vi "Reg Ref.vi"(7 "Tag":T1, 8 "error in (no error)":errorcluster caption="错误输入（无错误）", 11 "User Event Collection 输入":refnum<class "User Event Collection.lvclass"> caption="DNL_LabVIEW Object in") -> (0 "error out":errorcluster caption="错误输出", 2 "Event Registration Refnum":T2, 3 "User Event Collection 输出":refnum<class "User Event Collection.lvclass"> caption="DNL_LabVIEW Object out")   [LabVIEW 2013, in "User Event Collection.lvclass"]
uses:
  User Event Collection.lvclass
  <resource>/importtools/Common/Event/Data Type/Event Registeration Refnum.ctl
  Tag.ctl
  User Event Collection.lvclass/User Event Collection.ctl
  <resource>/importtools/Common/Event/NISAST Event.lvclass
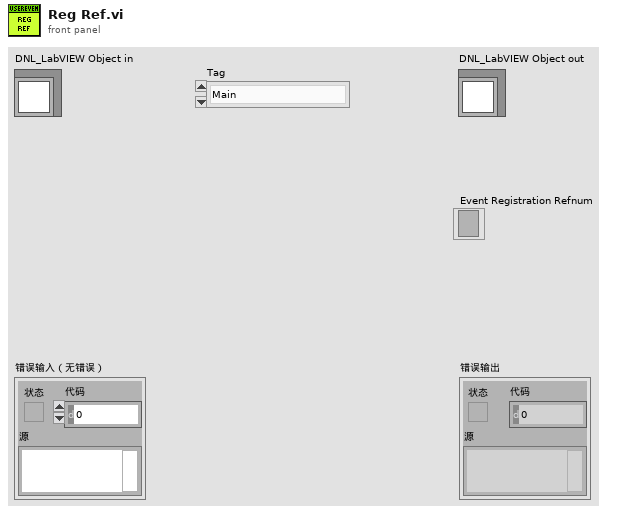
[diagram p1: front panel]
types:
  T1 = typedef "User Event Collection.lvclass/Tag.ctl" = enum16{"Main", "UI"}
  T2 = typedef "NISAST Event.lvclass/Event Registeration Refnum.ctl" = refnum<event-registration>
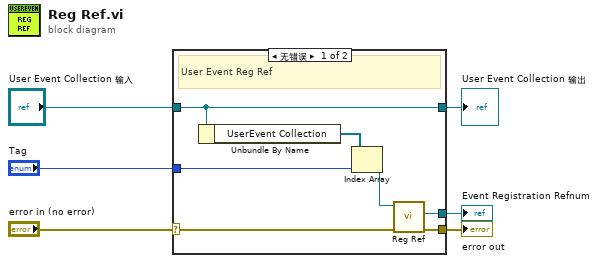
[diagram p0: block diagram]
diagram:
  n1 = case shown="无错误" "error in (no error)" {
    selector: "error in (no error)" -> [w8 w15]
    tunnel: [w7 w15] -> w5
    tunnel: [w13 w14] -> w3
    tunnel: "User Event Collection 输入" -> [w13 w14]
    tunnel: "Tag" -> [w11 _]
    tunnel: [w9 _] -> w1
    frame No Error {
      # "User Event Reg Ref"
      n2 = Unbundle By Name(w13) -> ("UserEvent Collection"=w12:refnum<class "NISAST Event.lvclass">[])
      n3 = Index Array(array=w12, index=w11) -> (element=w10:refnum<class "NISAST Event.lvclass">)
      n4 = call-dynamic "Reg Ref.vi"("error in (no error)"=w8, "Event in"=w10) -> ("error out"=w7:errorcluster, "Event Registration Refnum"=w9:T2)  [unwired: 7 in, 1 out]
    }
    frame Error {
    }
  }
  "error out" <- w5
  "User Event Collection 输出" <- w3
  "Event Registration Refnum" <- w1
